vi "Macro Text to Cluster.vi"(8 "Error In":errorcluster, 11 "Macro Text IN":string) -> (0 "Error Out":errorcluster, 3 "Macro Cluster Array OUT":T1[](array[typedef]))   [LabVIEW 2012]
uses:
  Custom Controls and Typedefs/Macro_CommandStruct.ctl
  Custom Controls and Typedefs/Macro_Action_List.ctl
  Custom Controls and Typedefs/Macro_ArgumentStruct.ctl
  <vilib>/regexp/Match Regular Expression.xnode
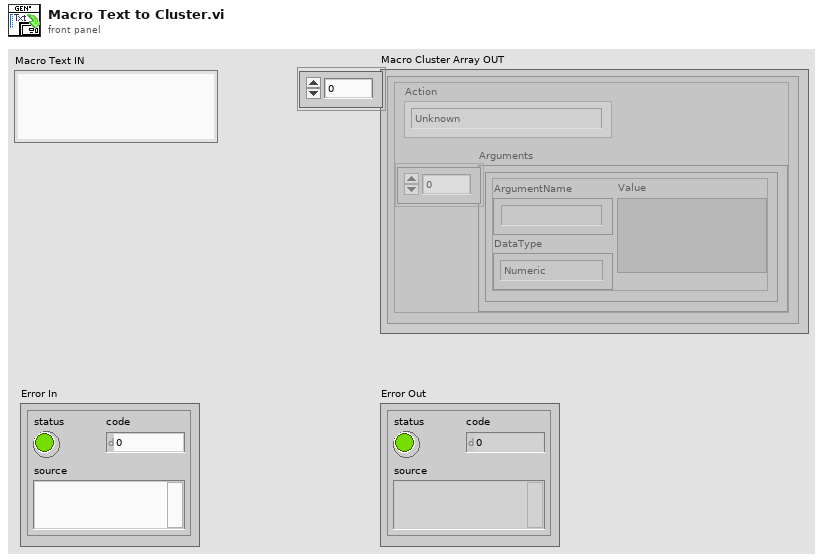
[diagram p1: front panel]
types:
  T1 = typedef "Macro_CommandStruct.ctl" = cluster{"Action":T2, "Arguments":T3[]}
  T2 = typedef "Macro_Action_List.ctl" = enum16{"Unknown", "2D.Frame.Scan", "2D.Line.Scan", "Load.Settings.File", "Move.To.Position", "Pause", "Z.Stack", "LOOP.Start", "LOOP.End"}
  T3 = typedef "Macro_ArgumentStruct.ctl" = cluster{"ArgumentName":string, "DataType":enum16{"Numeric", "String"}, "Value":variant}
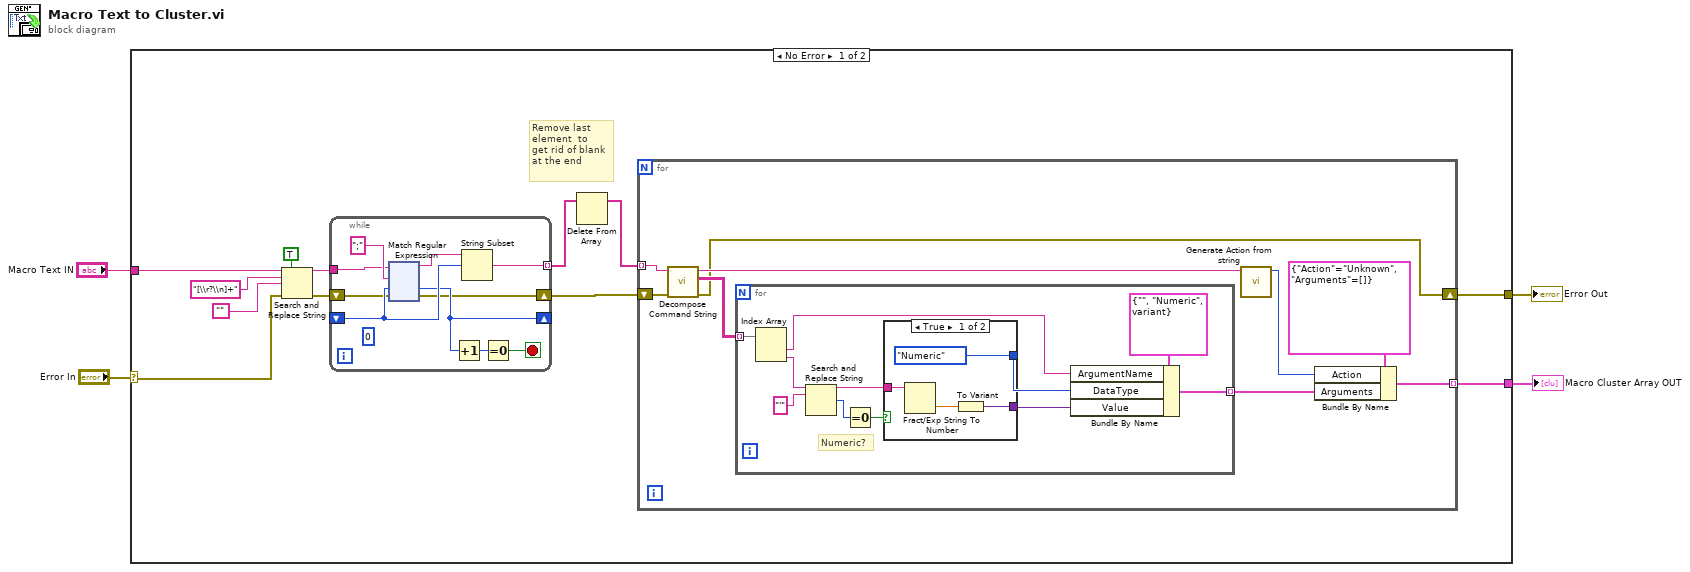
[diagram p0: block diagram]
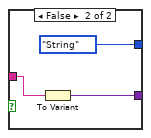
[diagram p2: hidden frame]
diagram:
  n1 = case shown="No Error" "Error In" {
    selector: "Error In" -> [w12 w165]
    tunnel: [w9 _] -> w3
    tunnel: [w8 w165] -> w2
    tunnel: "Macro Text IN" -> [w5 _]
    frame No Error {
      # "Remove last \nelement  to \nget rid of blank\nat the end"
      n2 = Search and Replace String(replace all?=TRUE ("replace all? (F)"), input string=w5, search string="[\\r?\\n]+", replace string="", error in=w12) -> (result string=w13:string, error out=w11:errorcluster)  [unwired: 3 in, 2 out]
      n3 = while {
        tunnel: w13 -> [w50]
        shift-right: [w46] -> _
        shift-left: _ -> [w47]
        tunnel: [w48] -> w7 mode=indexing
        shift-right: [w44] -> w10
        shift-left: w11 -> [w45]
        stop <- w53 stop-if-true
        (unwired) 0 ("offset of match")
        n4 = xnode "Match Regular Expression"("input string"=w50, "regular expression"=";" ("search string/char (-)"), "offset (0)"=w47, "error in"=w45) -> ("before match"=w49:string, "offset past match"=w46:i32, "error out"=w44:errorcluster)  [unwired: 2 in, 2 out]
        n5 = Increment(x=w46) -> (x+1=w52:i32)
        n6 = String Subset(string=w49, offset (0)=w47) -> (substring=w48:string)  [unwired: 1 in]
        n7 = Equal To 0?(x=w52) -> (x = 0?=w53:bool)
      }
      n8 = Delete From Array(array=w7) -> (array with subset deleted=w6:string[])  [unwired: 2 in, 1 out]
      n9 = for {
        tunnel: w6 -> [w25] mode=indexing
        tunnel: [w18] -> w9 mode=indexing
        shift-right: [w17] -> w8
        shift-left: w10 -> [w24]
        n10 = call "Decompose Command String.vi"("Error In"=w24, "Command IN"=w25) -> ("Error Out"=w17:errorcluster, "ArgumentTable"=w23:string[][], "Action"=w21:string)  [unwired: 7 in]
        n11 = for {
          tunnel: w23 -> [w35] mode=indexing
          tunnel: [w26] -> w19 mode=indexing
          # "Numeric?"
          n12 = Index Array(array=w35) -> (element #1=w34:string, element #2=w29:string)  [unwired: 2 in]
          n13 = Search and Replace String(input string=w29, search string="'") -> (result string=w30:string, number of replacements=w32:i32)  [unwired: 6 in, 2 out]
          n14 = Equal To 0?(x=w32) -> (x = 0?=w31:bool)
          n15 = case shown="True" w31 {
            tunnel: w30 -> [w40 w43]
            tunnel: [enum16{"Numeric", "String"}."Numeric" ("DataType") enum16{"Numeric", "String"}."String" ("DataType")] -> w28
            tunnel: [w37 w41] -> w27
            frame True {
              n16 = Fract/Exp String To Number(string=w40) -> (number=w39:dbl)  [unwired: 3 in, 1 out]
              n17 = To Variant(anything=w39) -> (Variant=w37:variant)
            }
            frame False {
              n18 = To Variant(anything=w43) -> (Variant=w41:variant)
            }
          }
          n19 = Bundle By Name(cluster=T3 {"ArgumentName"="", "DataType"=enum."Numeric", "Value"=variant} ("Argument"), "ArgumentName"=w34, "DataType"=w28, "Value"=w27) -> (w26:T3)
        }
        n20 = call "Generate Action from string.vi"("Command Text"=w21) -> ("Action"=w20:T2)  [unwired: 9 in, 1 out]
        n21 = Bundle By Name(cluster=T1 {"Action"=enum."Unknown", "Arguments"=[]} ("Macro Commands"), "Action"=w20, "Arguments"=w19) -> (w18:T1)
      }
    }
    frame Error {
    }
  }
  "Error Out" <- w2
  "Macro Cluster Array OUT" <- w3
